vi "Get JSON setup.vi"(8 "error in (no error)":errorcluster, 11 "Interface in":refnum<class "Interface.lvclass">) -> (0 "error out":errorcluster, 3 "Interface out":refnum<class "Interface.lvclass">)   [LabVIEW 2018, in "Interface.lvclass"]
uses:
  Interface.lvclass
  Interface.lvclass/Interface.ctl
  JSON/JSON.lvclass/JSON.ctl
  JSON/JSON.lvclass
panel:
  in  "Camera Setup":T1={"t_exp"=1e-05, "hss"=0, "preamp"=0, "sub_img"=1, "bin"=1, "em_gain"=2.0, "em_mode"="", "kinetic_series_length"=1, "img_name"="", "obs_type"="", "output"=0.0, "star_radius"=0.0, "obj_coords"=""} {"kinetic_series_length" min=1; "em_gain" min=2.0 max=300.0; "bin" min=1 max=2; "sub_img" min=1 max=1024; "preamp" items=["Gain 1", "Gain 2"]; "hss" items=["30 MHz", "20 MHz", "10 MHz", "  1 MHz"]; "t_exp" min=1e-05}
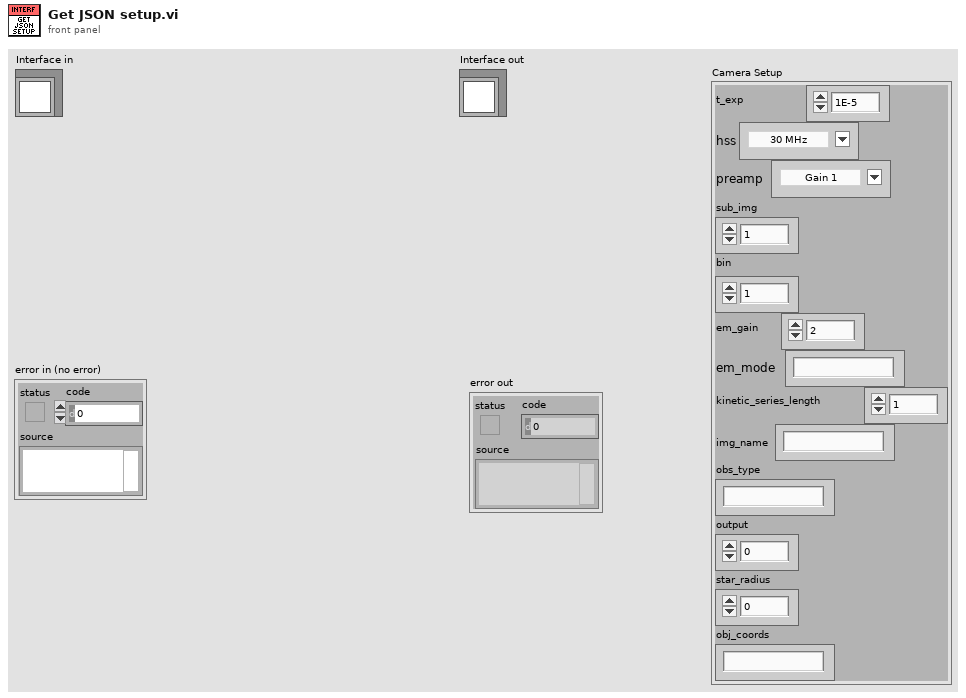
[diagram p1: front panel]
types:
  T1 = cluster{"t_exp":dbl, "hss":u8, "preamp":u8, "sub_img":u16, "bin":u8, "em_gain":dbl, "em_mode":string, "kinetic_series_length":u16, "img_name":string, "obs_type":string, "output":dbl, "star_radius":dbl, "obj_coords":string}
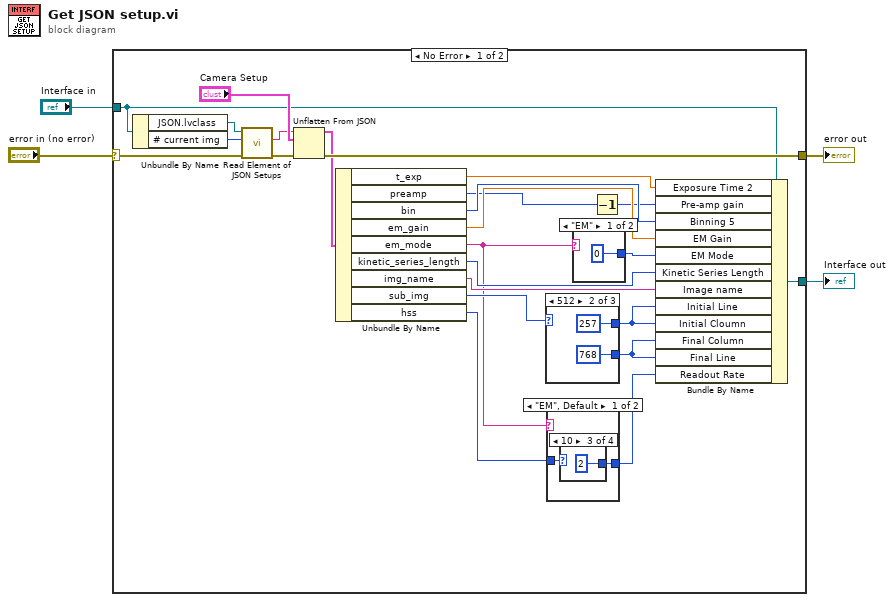
[diagram p0: block diagram]
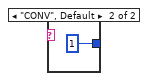
[diagram p2: hidden frame]
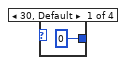
[diagram p3: hidden frame]
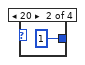
[diagram p4: hidden frame]
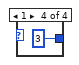
[diagram p5: hidden frame]
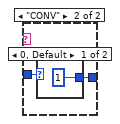
[diagram p6: hidden frame]
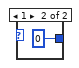
[diagram p7: hidden frame]
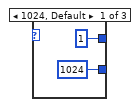
[diagram p8: hidden frame]
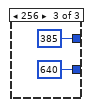
[diagram p9: hidden frame]
diagram:
  n1 = case shown="No Error" "error in (no error)" {
    selector: "error in (no error)" -> [w27 w48]
    tunnel: [w25 w48] -> w3
    tunnel: [w21 w47] -> w1
    tunnel: "Interface in" -> [w22 w47]
    frame No Error {
      n2 = Unbundle By Name(w22) -> ("JSON.lvclass"=w28:refnum<class "JSON.lvclass">, "# current img"=w16:u16)
      n3 = call "Read Element of JSON Setups.vi"("error in (no error)"=w27, "index"=w16, "JSON in"=w28) -> ("error out"=w26:errorcluster, "String"=w5:string)  [unwired: 6 in, 1 out]
      n4 = Unflatten From JSON(JSON string=w5, type and defaults="Camera Setup", error in (no error)=w26) -> (value=w23:T1, error out=w25:errorcluster)  [unwired: 4 in]
      n5 = Unbundle By Name(w23) -> ("t_exp"=w20:dbl, "preamp"=w7:u8, "bin"=w18:u8, "em_gain"=w19:dbl, "em_mode"=w9:string, "kinetic_series_length"=w17:u16, "img_name"=w15:string, "sub_img"=w14:u16, "hss"=w11:u8)
      n6 = case shown="512" w14 {
        tunnel: [1 257 385] -> w13
        tunnel: [1024 768 640] -> w12
        frame 1024, Default {
        }
        frame 512 {
        }
        frame 256 {
        }
      }
      n7 = case shown="\"EM\", Default" w9 {
        tunnel: w11 -> [w31 w38]
        tunnel: [w32 w37] -> w8
        frame "EM", Default {
          n8 = case shown="10" w31 {
            tunnel: [0 1 2 3] -> w32
            frame 30, Default {
            }
            frame 20 {
            }
            frame 10 {
            }
            frame 1 {
            }
          }
        }
        frame "CONV" {
          n9 = case shown="0, Default" w38 {
            tunnel: [1 0] -> w37
            frame 0, Default {
            }
            frame 1 {
            }
          }
        }
      }
      n10 = case shown="\"EM\"" w9 {
        tunnel: [0 1] -> w10
        frame "EM" {
        }
        frame "CONV", Default {
        }
      }
      n11 = Decrement(x=w7) -> (x-1=w6:u8)
      n12 = Bundle By Name(cluster=w22, "Exposure Time 2"=w20, "Pre-amp gain"=w6, "Binning 5"=w18, "EM Gain"=w19, "EM Mode"=w10, "Kinetic Series Length"=w17, "Image name"=w15, "Initial Line"=w13, "Initial Cloumn"=w13, "Final Column"=w12, "Final Line"=w12, "Readout Rate"=w8) -> (w21:refnum<class "Interface.lvclass">)
    }
    frame Error {
    }
  }
  "error out" <- w3
  "Interface out" <- w1
